vi "configureTrigger_action.vi"(0 "HGF_AVT_F033B":refnum<class "HGF_AVT_F033B.lvclass">, 1 "Type":u32(ring) items=["External"=0, "RTSI"=1, "ISO In"=2, "Scaled Encoder"=5, "Software Trigger"=6], 2 "Line Number":u32, 3 "Frame timeout (ms)":u32=1000, 4 "Action":u32(ring) items=["Disabled", "Trigger start of acquisition", "Trigger start of each buffer list", "Trigger each buffer", "Trigger each line (linescan)", "Trigger end of acquisition"], 5 "error in (no error)":errorcluster, 6 "Activation":u32(ring) items=["Rising Edge", "Falling Edge", "AnyEdge", "LevelHigh", "LevelLow"], 7 "Delay":cluster{"Value":dbl, "Units":u32}={"Value"=0.0, "Units"=5} {"Units" items=["Scaled Encoder Counts"=4, "Milliseconds"=5]}, 8 "Mode":T1(ring), 9 "Skip trigger (linescan only)":u32) -> (14 "dup HGF_AVT_F033B":refnum<class "HGF_AVT_F033B.lvclass">, 19 "error out":errorcluster)   [LabVIEW 2014, in "HGF_IMAQ.lvlib" / "HGF_AVT_F033B.lvclass"]
doc: "Configures the trigger conditions for an acquisition. Use this VI before any acquisition VI to setup a triggered image acquisition."
uses:
  HGF_AVT_F033B.lvclass
  HGF_VisionTools/HGF_VisionTools.lvlib
  HGF_VisionTools/IMAQdx_setAttribute_Enum.vi
  HGF_Auxiliary/ErrorCode.ctl
  HGF_Auxiliary/HGF_Auxiliary.lvlib
  HGF_Auxiliary/Severity.ctl
  HGF_ImaqDx/HGF_ImaqDx.lvclass
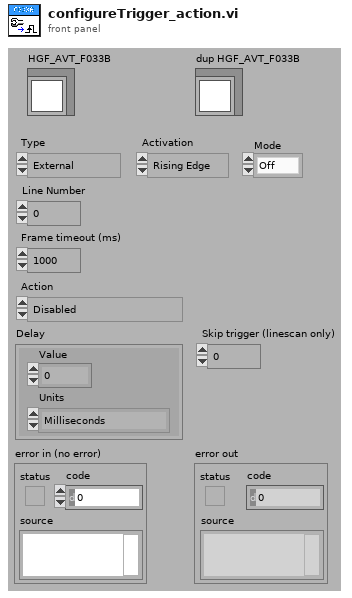
[diagram p1: front panel]
types:
  T1 = enum16{"Off", "Mode 0", "Mode 1", "Mode 2", "Mode 3", "Mode 4", "Mode 5"}
  T2 = typedef "HGF_Auxiliary.lvlib/Severity.ctl" = enum16{"Info", "Warning", "Fault", "Error", "Fatal"}
  T3 = typedef "HGF_Auxiliary.lvlib/ErrorCode.ctl" = enum32{"No error", "Function not supported.", "This VI is for friends only.", "Reference object aready exisits.", "Parameter out of range.", "Not a rendezvous.", "Invalid notifier reference.", "Invalid queue reference.", "Self-Test not supported.", "Reset not supported.", "IDN query not supported.", "Error query not supported.", "Incorrect addressee.", "Object already exists.", "No class name specified", "Driver not supported", "Attribute is not writable"}
  T4 = typedef "IMAQdx.ctl" = refnum<k21>
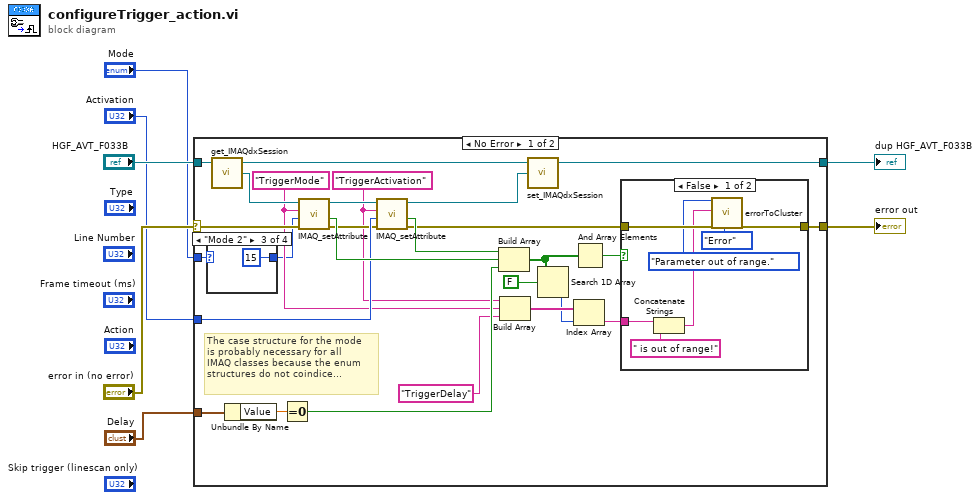
[diagram p0: block diagram]
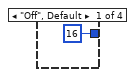
[diagram p2: hidden frame]
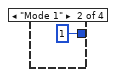
[diagram p3: hidden frame]
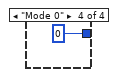
[diagram p4: hidden frame]
diagram:
  n1 = case shown="No Error" "error in (no error)" {
    selector: "error in (no error)" -> [w34 w47]
    tunnel: "HGF_AVT_F033B" -> [w28 w48]
    tunnel: [w31 w47] -> w6
    tunnel: [w26 w48] -> w5
    tunnel: "Activation" -> [w30 _]
    tunnel: "Mode" -> [w9 _]
    tunnel: "Delay" -> [w23 _]
    frame No Error {
      w13 = "TriggerActivation" ("Attribute Name")
      w12 = "TriggerMode" ("Attribute Name")
      # "The case structure for the mode\nis probably necessary for all\nIMAQ classes because the enum\nstructures do not coindice..."
      n2 = case shown="\"Mode 2\"" w9 {
        tunnel: [16 1 15 0] -> w8
        frame "Off", Default {
        }
        frame "Mode 1" {
        }
        frame "Mode 2" {
        }
        frame "Mode 0" {
        }
      }
      n3 = call "get_IMAQdxSession.vi"("HGF_ImaqDx in"=w28) -> ("IMAQdx Session"=w29:T4, "HGF_ImaqDx out"=w27:refnum<class "HGF_AVT_F033B.lvclass">)  [unwired: 2 in, 1 out]
      n4 = Unbundle By Name(w23) -> ("Value"=w22:dbl)
      n5 = Equal To 0?(x=w22) -> (x = 0?=w21:bool)
      n6 = call-poly "IMAQ_setAttribute.vi"("error in (no error)"=w34, "Value (Enum)"=w8, "Attribute Name"=w12, "IMAQdx Session"=w29) -> ("error out"=w24:errorcluster, "In Range?"=w32:bool, "dup IMAQdx Session"=w25:T4)  [unwired: 1 in]
      n7 = call-poly "IMAQ_setAttribute.vi"("error in (no error)"=w24, "Value (Enum)"=w30, "Attribute Name"=w13, "IMAQdx Session"=w25) -> ("error out"=w10:errorcluster, "In Range?"=w33:bool, "dup IMAQdx Session"=w11:T4)  [unwired: 1 in]
      n8 = Build Array(w33, w32, w21) -> (w19:bool[])
      n9 = Build Array(w13, w12, "TriggerDelay" ("element")) -> (w17:string[])
      n10 = call "set_IMAQdxSession.vi"("IMAQdx Session"=w11, "HGF_ImaqDx in"=w27) -> ("HGF_ImaqDx out"=w26:refnum<class "HGF_AVT_F033B.lvclass">)  [unwired: 2 in, 1 out]
      n11 = Search 1D Array(1D array=w19, element=FALSE) -> (index of element=w16:i32)  [unwired: 1 in]
      n12 = Index Array(array=w17, index=w16) -> (element=w14:string)
      n13 = And Array Elements(Boolean array=w19) -> (logical AND=w20:bool)
      n14 = case shown="False" w20 {
        tunnel: w10 -> [w45 w46]
        tunnel: [w44 w46] -> w31
        tunnel: w14 -> [w40 _]
        frame False {
          n15 = Concatenate Strings(w40, " is out of range!" ("string")) -> (w39:string)
          n16 = call "errorToCluster.vi"("error code"=ErrorCode."Parameter out of range.", "error message (\"\")"=w39, "error in (no error)"=w45, "severity (Error)"=Severity."Error") -> ("error out"=w44:errorcluster)  [unwired: 15 in]
        }
        frame True {
        }
      }
    }
    frame Error {
    }
  }
  "error out" <- w6
  "dup HGF_AVT_F033B" <- w5
